vi "Overcome Static Friction.vi"(1 "lower limit":dbl=0.3 format="%#_13g", 2 "x":dbl) -> (0 "x*y":dbl)   [LabVIEW 2020]
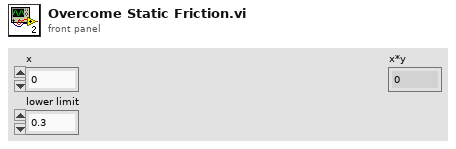
[diagram p1: front panel]
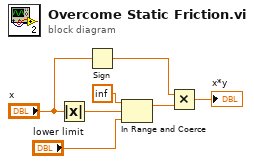
[diagram p0: block diagram]
diagram:
  n1 = Absolute Value(x="x") -> (abs(x)=w5:dbl)
  n2 = Sign(1:"x") -> (0:w2:dbl)
  n3 = In Range and Coerce(upper limit=inf, x=w5, lower limit="lower limit") -> (coerced(x)=w3:dbl)  [unwired: 1 out]
  n4 = Multiply(x=w2, y=w3) -> (x*y=→"x*y":dbl)
